vi "testing.vi"() -> ()   [LabVIEW 2021]
uses:
  <vilib>/rvi/Emulation/niFpgaGetClockAttributes.vi
  <vilib>/rvi/Emulation/niFpgaSctlEmulationGetInTimedLoop.vi
  <vilib>/rvi/Emulation/niFpgaEmulationReportErrorSimple.vi
  <vilib>/rvi/Emulation/niFpgaCriticalErrorInLSC.vi
panel:
  out "sine B":i16
  out "sine C":i16
  out "sine A":i16
  out "square wave out":i16 caption="sawtooth wave out\nfixed constant"
  out "Wave A":i16(graph)
  in  "Count(mSec)":u32
  out "Wave B":i16(graph)
  out "Wave C":i16(graph)
  out "All 3 Waves":i16[](graph)
  out "D03":bool
  out "D02":bool
  out "D04":bool
  out "d01":bool
  out "D00":bool
  out "D05":bool
  out "SawTooth":i16(graph)
  out "for loop index 2":i32
  in  "stop":bool
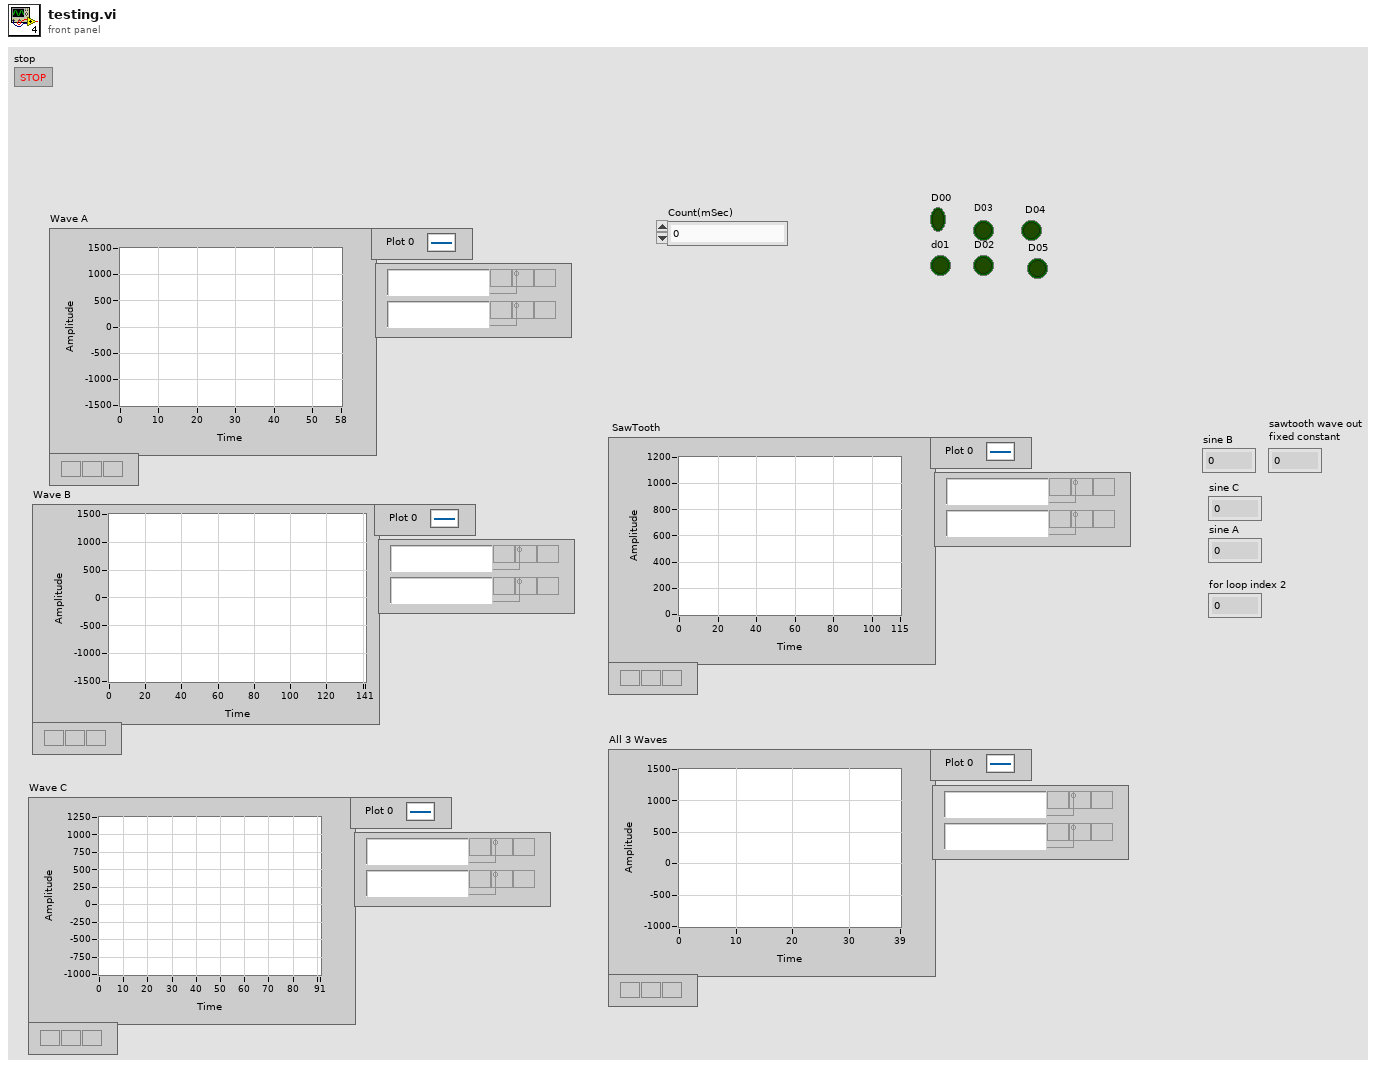
[diagram p1: front panel]
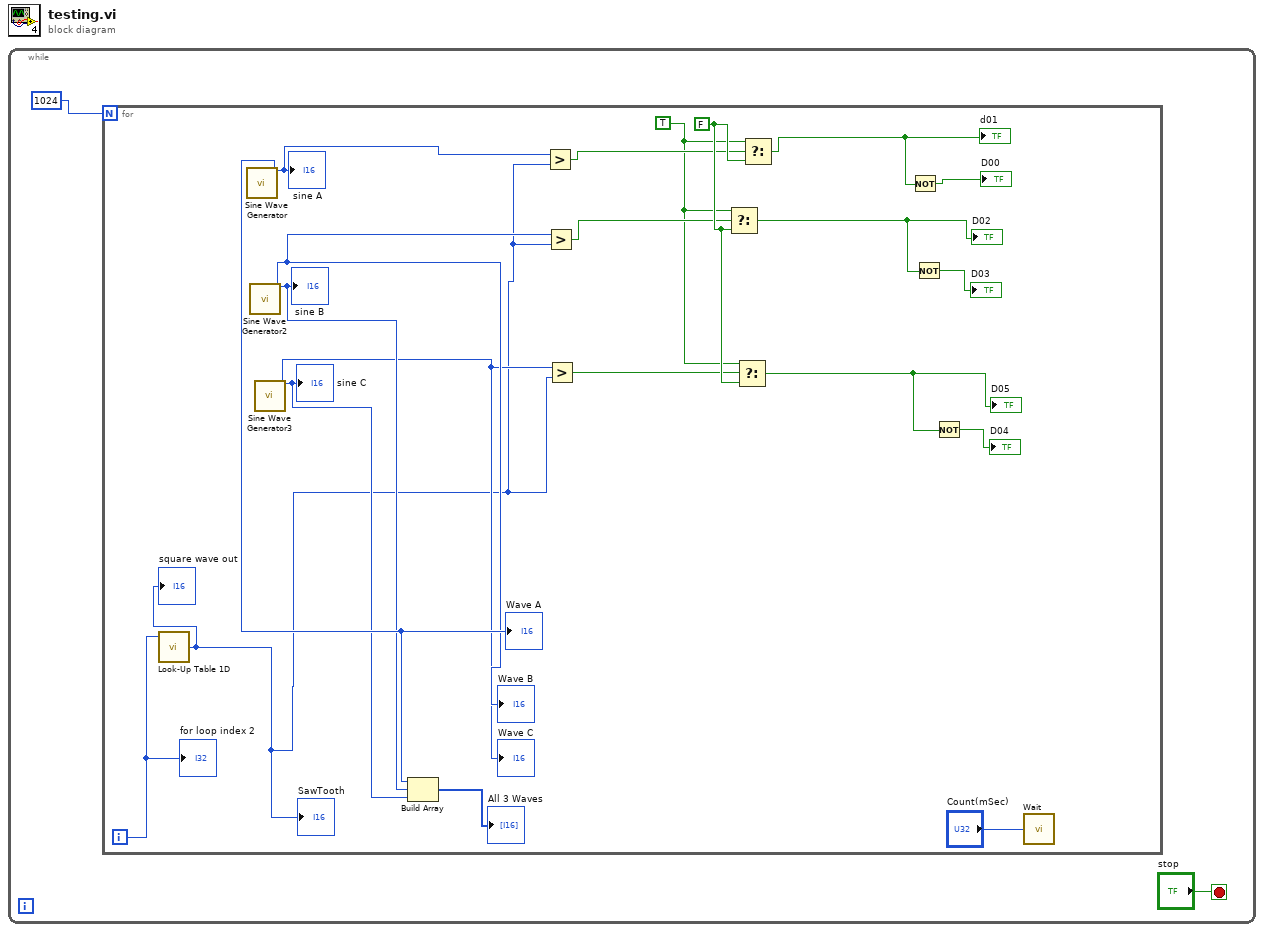
[diagram p0: block diagram]
diagram:
  n1 = while {
    stop <- "stop" stop-if-true
    n2 = for {
      N: 1024 -> [_]
      i -> [w3]
      w18 = FALSE
      w5 = TRUE
      n3 = call "Look-Up Table 1D"("address"=w3) -> ("data out"=w4:i16)  [unwired: 8 in]
      "square wave out" <- w4
      "SawTooth" <- w4
      n4 = call "Sine Wave Generator"() -> ("sine out"=w8:i16)  [unwired: 14 in, 1 out]
      "sine A" <- w8
      "Wave A" <- w8
      n5 = call "Sine Wave Generator2"() -> ("sine out"=w7:i16)  [unwired: 14 in, 1 out]
      "sine B" <- w7
      "Wave B" <- w7
      n6 = call "Sine Wave Generator3"() -> ("sine out"=w6:i16)  [unwired: 14 in, 1 out]
      "sine C" <- w6
      "Wave C" <- w6
      n7 = Build Array(w8, w7, w6) -> (→"All 3 Waves":i16[])
      n8 = Greater?(x=w8, y=w4) -> (0:w15:bool)
      n9 = Greater?(x=w7, y=w4) -> (0:w16:bool)
      n10 = Greater?(x=w6, y=w4) -> (0:w17:bool)
      n11 = Select(t=w5, s=w16, f=w18) -> (s? t:f=w10:bool)
      "D02" <- w10
      n12 = Select(t=w5, s=w17, f=w18) -> (s? t:f=w12:bool)
      "D05" <- w12
      n13 = Select(t=w5, s=w15, f=w18) -> (s? t:f=w14:bool)
      "d01" <- w14
      n14 = Not(x=w14) -> (.not. x?=→"D00":bool)
      n15 = Not(x=w10) -> (.not. x?=→"D03":bool)
      n16 = Not(x=w12) -> (.not. x?=→"D04":bool)
      n17 = call "Wait"("Count(uSec)"="Count(mSec)") -> ()  [unwired: 1 out]
      "for loop index 2" <- w3
    }
  }
